vi "KundtsImpulse.vi"() -> ()   [LabVIEW 2014]
uses:
  <vilib>/Analysis/2dsp.llb/Real FFT.vi
  <vilib>/Analysis/NI_AALPro.lvlib
panel:
  out "XY Graph":cluster{dbl[], dbl[]}(graph)
  in  "error in":errorcluster
  out "error out":errorcluster
  out "FFT":dbl[](graph)
  in  "?":bool
  in  "Time (s)":dbl
  in  "Rate":dbl
  in  "Averages":dbl
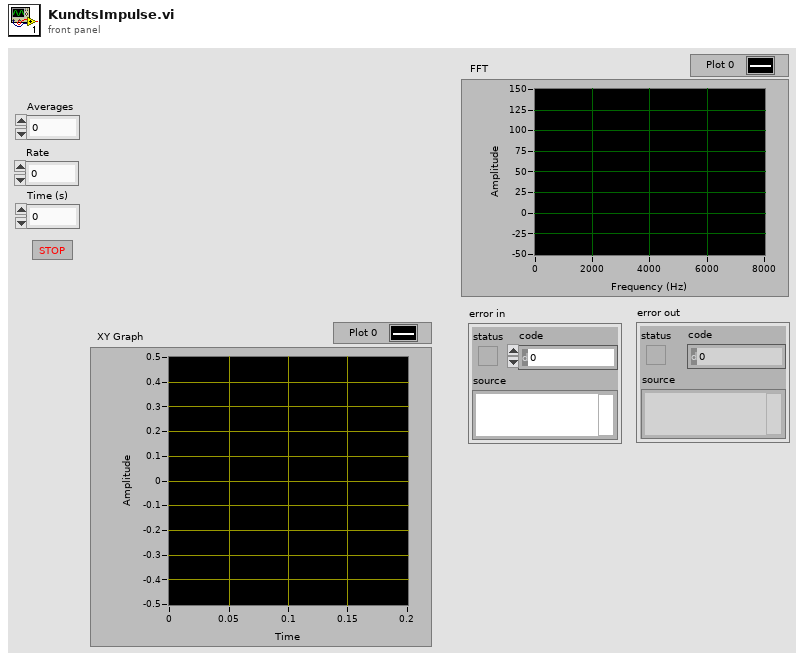
[diagram p1: front panel]
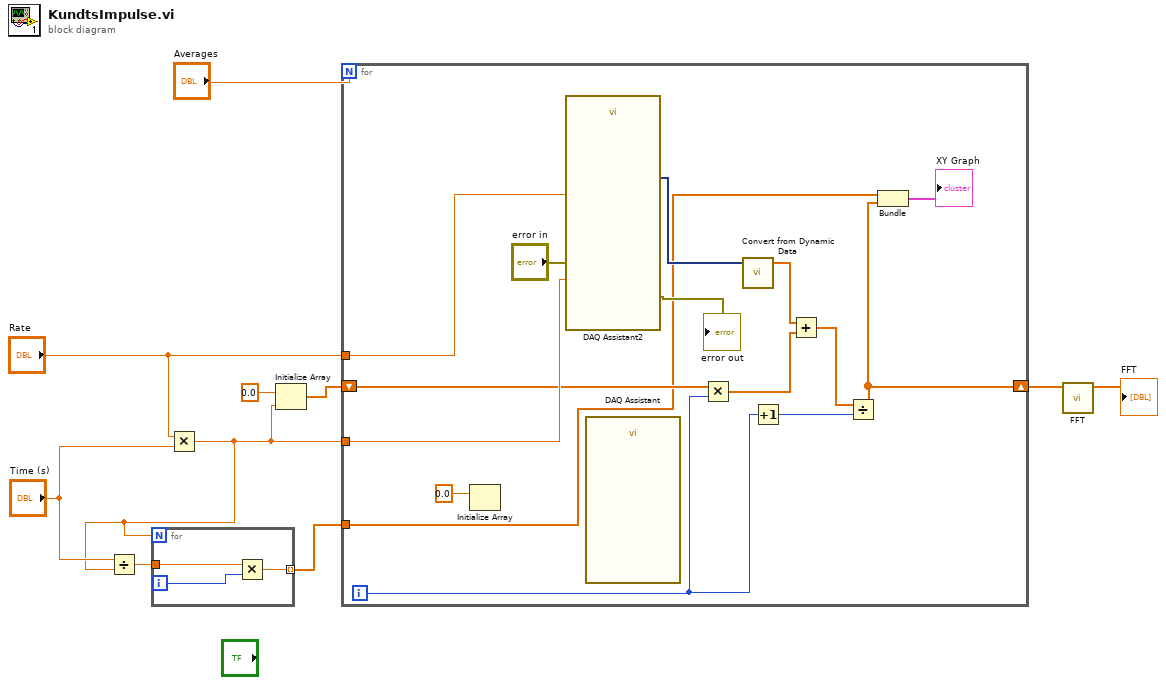
[diagram p0: block diagram]
diagram:
  n1 = Multiply(x="Rate", y="Time (s)") -> (x*y=w3:dbl)
  n2 = Divide(x="Time (s)", y=w3) -> (x/y=w2:dbl)
  n3 = for {
    N: w3 -> [_]
    tunnel: w2 -> [w13]
    tunnel: [w11] -> w1 mode=indexing
    i -> [w12]
    n4 = Multiply(x=w13, y=w12) -> (x*y=w11:dbl)
  }
  n5 = Initialize Array(0.0 ("element"), w3) -> (w8:dbl[])
  n6 = for {
    N: "Averages" -> [_]
    tunnel: "Rate" -> [w28]
    tunnel: w3 -> [w27]
    shift-right: [w15] -> w6
    shift-left: w8 -> [w26]
    tunnel: w1 -> [w16]
    i -> [w21]
    n7 = Initialize Array(0.0 ("element")) -> ()  [unwired: 1 in, 1 out]
    n8 = call "DAQ Assistant2"("rate"=w28, "number of samples"=w27, "error in"="error in") -> ("data"=w25:dynamicdata, "error out"=→"error out":errorcluster)  [unwired: 14 in, 1 out]
    n9 = call "DAQ Assistant"() -> ()  [unwired: 18 in, 2 out]
    n10 = Multiply(x=w26, y=w21) -> (x*y=w24:dbl[])
    n11 = call "Convert from Dynamic Data"("Dynamic Data Type"=w25) -> ("Array"=w23:dbl[])  [unwired: 3 in]
    n12 = Increment(x=w21) -> (x+1=w20:i32)
    n13 = Add(x=w23, y=w24) -> (x+y=w22:dbl[])
    n14 = Divide(x=w22, y=w20) -> (x/y=w15:dbl[])
    n15 = Bundle(w16, w15) -> (→"XY Graph":cluster{dbl[], dbl[]})  [unwired: 1 in]
  }
  n16 = call-poly <vilib>:"FFT.vi"("X"=w6) -> ("FFT {X}"=→"FFT":cdb[])  [unwired: 9 in, 1 out]
